vi "Crab.vi"   [LabVIEW 2020]
uses:
  Robot Global Data.vi
  <vilib>/addons/control/pid/pid.llb/PID (DBL).vi
  <vilib>/addons/control/pid/NI_PID_pid.lvlib
panel:
  # "p=0.014"
types:
  T1 = cluster{"proportional gain (Kc)":dbl, "integral time (Ti, min)":dbl, "derivative time (Td, min)":dbl}
  T2 = typedef "WPI_MotorControlDeviceRef.ctl" = cluster{"DeviceStatus":errorcluster, "Type":T3, "PWM":cluster{"PWM Channel":T4, "DeadBand":T5}, "CAN":cluster{"Device Number":u8, "SetOutput VI Ref":variant, "GetOutput VI Ref":variant, "Enable VI Ref":variant, "Disable VI Ref":variant, "Data":variant}, "Invert":bool, "DIO PWM":cluster{"PWM \"Enable\" Channel":T4, "DIOChannel":T6, "PWM Rate":dbl}}
  T3 = typedef "WPI_MotorControlType.ctl" = enum16{"PWM", "CAN", "DIO PWM"}
  T4 = typedef "FPGA_DIOPWMChannel.ctl" = enum8{"PWM 0", "PWM 1", "PWM 2", "PWM 3", "PWM 4", "PWM 5", "PWM 6", "PWM 7", "PWM 8", "PWM 9", "PWM MXP 0", "PWM MXP 1", "PWM MXP 2", "PWM MXP 3", "PWM MXP 4", "PWM MXP 5", "PWM MXP 6", "PWM MXP 7", "PWM MXP 8", "PWM MXP 9", "Invalid"}
  T5 = typedef "WPI_PWMDeadband.ctl" = cluster{"Name":string, "maxPositivePwm":i32, "minPositivePwm":i32, "centerPwm":i32, "maxNegativePwm":i32, "minNegativePwm":i32, "angularRange":u16}
  T6 = typedef "FPGA_DIOChannel.ctl" = enum8{"DIO 0", "DIO 1", "DIO 2", "DIO 3", "DIO 4", "DIO 5", "DIO 6", "DIO 7", "DIO 8", "DIO 9", "DIO MXP 0", "DIO MXP 1", "DIO MXP 2", "DIO MXP 3", "DIO MXP 4", "DIO MXP 5", "DIO MXP 6", "DIO MXP 7", "DIO MXP 8", "DIO MXP 9", "DIO MXP 10", "DIO MXP 11", "DIO MXP 12", "DIO MXP 13", "DIO MXP 14", "DIO MXP 15", "SPI Port CS1", "SPI Port CS2", "SPI Port CS3", "SPI Port MISO", "SPI Port MOSI", "Invalid"}
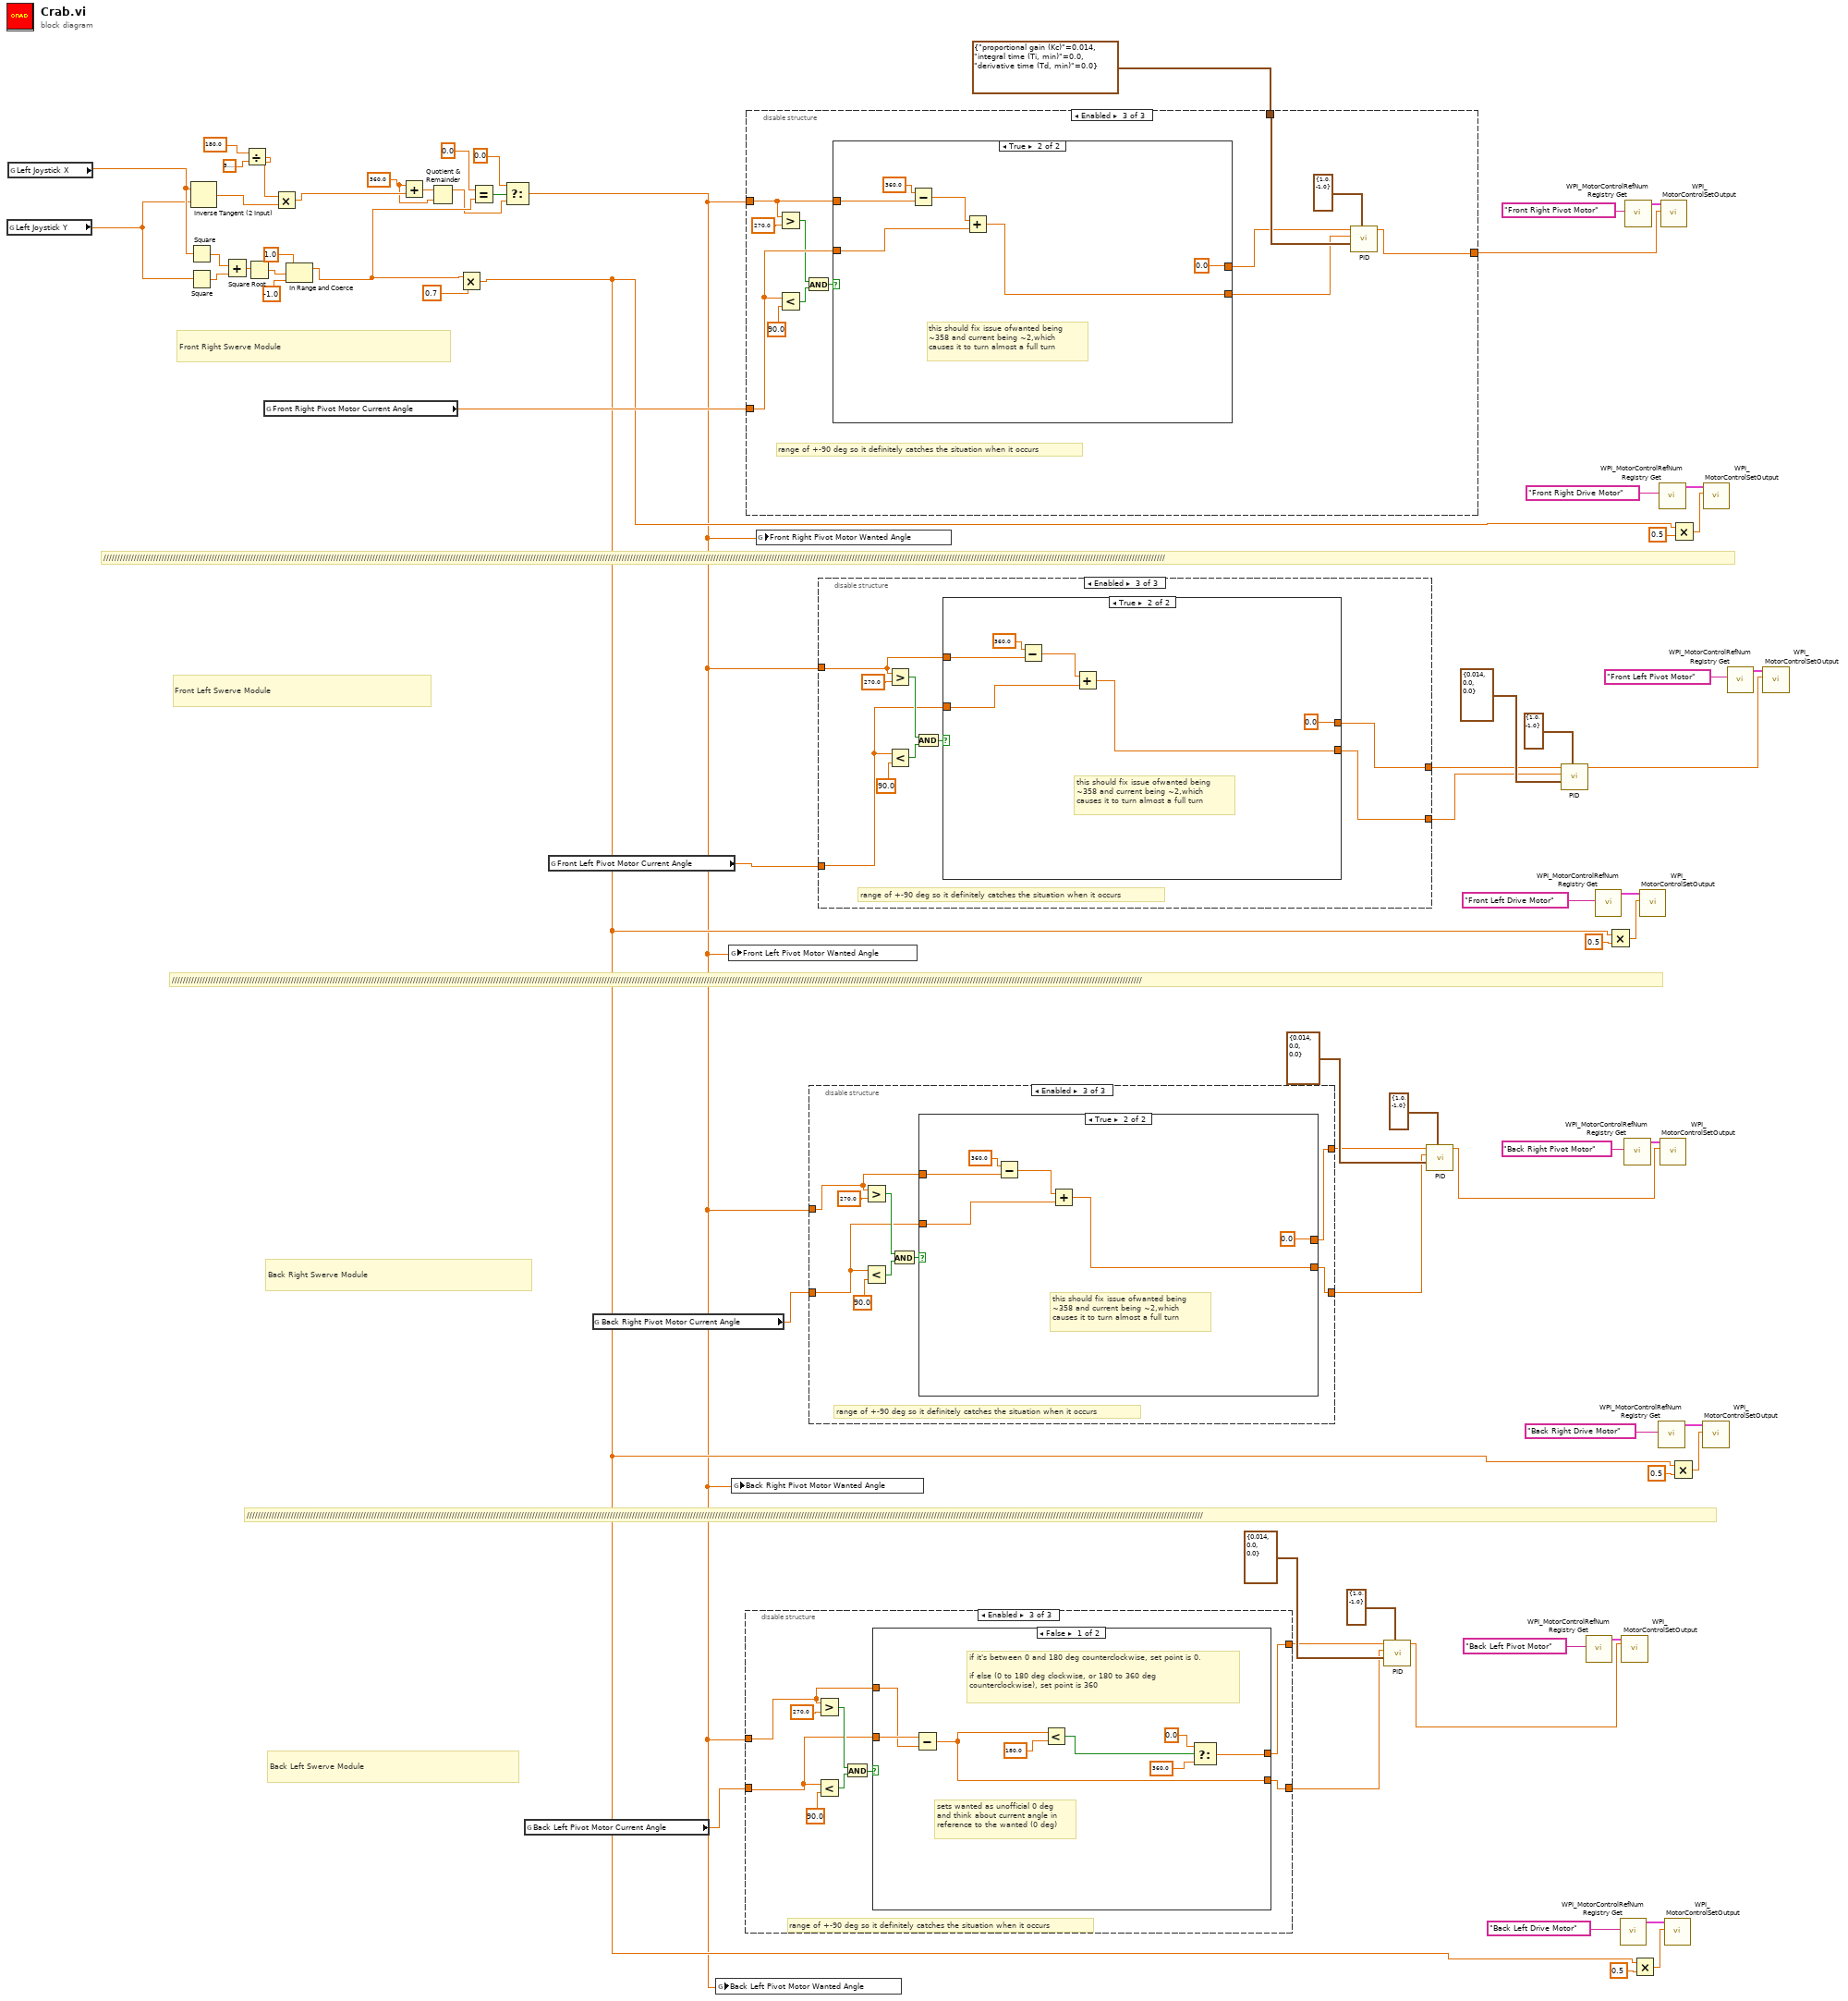
[diagram p0: block diagram]
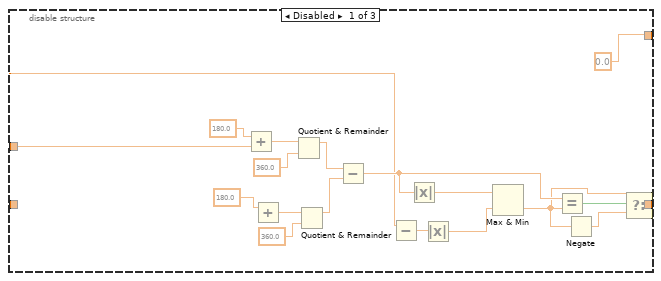
[diagram p2: hidden frame]
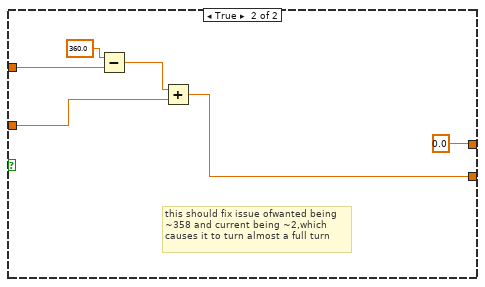
[diagram p4: hidden frame]
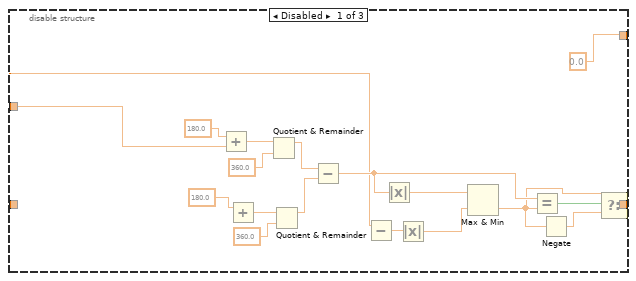
[diagram p5: hidden frame]
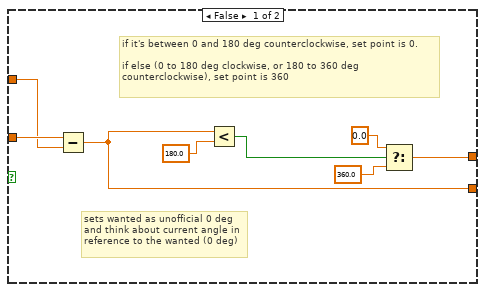
[diagram p7: hidden frame]
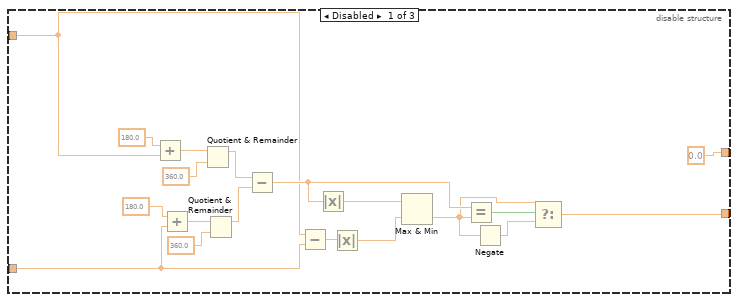
[diagram p8: hidden frame]
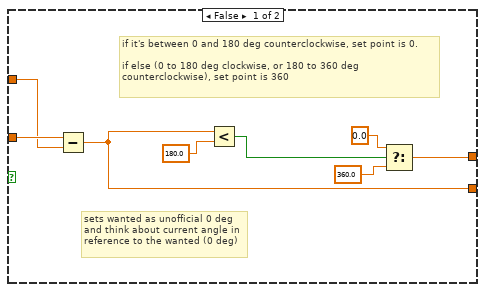
[diagram p10: hidden frame]
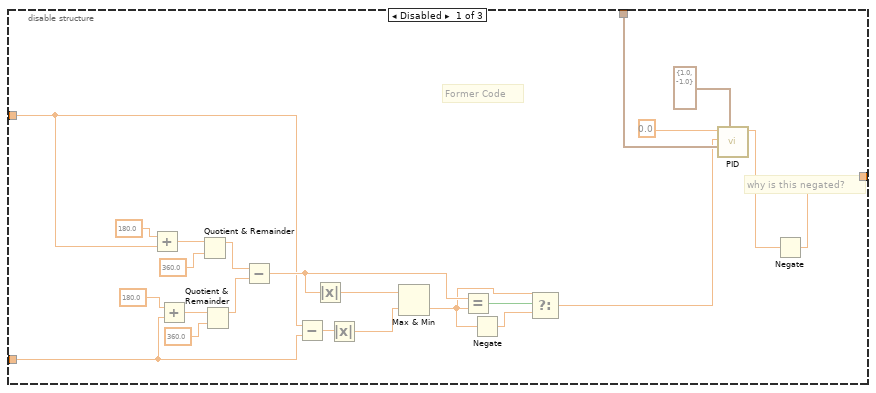
[diagram p11: hidden frame]
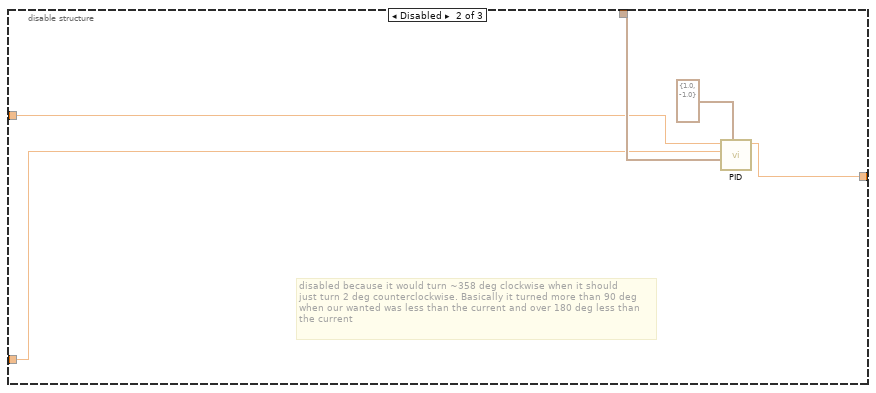
[diagram p12: hidden frame]
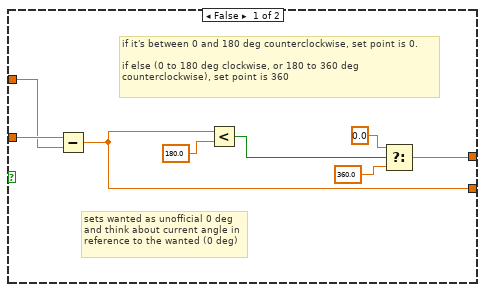
[diagram p13: hidden frame]
diagram:
  w60 = 360.0
  # "Back Left Swerve Module"
  # "/////////////////////////////////////////////////////////////////////////////////////////////////////////////////////////////////////////////////////////////////////////////////////////////////////////////////////////////////////////////////////////////////////////////////////////////////////////////////////////////////////////////////////////"
  # "//////////////////////////////////////////////////////////////////////////////////////////////////////////////////////////////////////////////////////////////////////////////////////////////////////////////////////////////////////////////////////////////////////////////////////////////////////////////////////////////////////////////////////////////"
  # "///////////////////////////////////////////////////////////////////////////////////////////////////////////////////////////////////////////////////////////////////////////////////////////////////////////////////////////////////////////////////////////////////////////////////////////////////////////////////////////////////////////////////////////////////////////////////////////////"
  # "Back Right Swerve Module"
  # "Front Left Swerve Module"
  # "Front Right Swerve Module"
  n1 = global read "Robot Global Data.vi" "Left Joystick Y"() -> (w50:dbl)
  n2 = global read "Robot Global Data.vi" "Left Joystick X"() -> (w51:dbl)
  n3 = Square(x=w51) -> (x^2=w57:dbl)
  n4 = Square(x=w50) -> (x^2=w56:dbl)
  n5 = Inverse Tangent (2 Input)(1:w50, 2:w51) -> (0:w55:dbl)
  n6 = Add(x=w57, y=w56) -> (x+y=w58:dbl)
  n7 = Divide(x=180.0, y=3.141592653589793) -> (x/y=w54:dbl)
  n8 = Square Root(x=w58) -> (sqrt(x)=w63:dbl)
  n9 = global read "Robot Global Data.vi" "Front Right Pivot Motor Current Angle"() -> (w26:dbl)
  n10 = Multiply(x=w54, y=w55) -> (x*y=w61:dbl)
  n11 = In Range and Coerce(upper limit=1.0, x=w63, lower limit=-1.0 ("upper limit")) -> (coerced(x)=w31:dbl)  [unwired: 1 out]
  n12 = Add(x=w60, y=w61) -> (x+y=w59:dbl)
  n13 = Quotient & Remainder(x=w59, y=w60) -> (x-y*floor(x/y)=w5:dbl)  [unwired: 1 out]
  n14 = Multiply(x=w31, y=0.7) -> (x*y=w6:dbl)
  n15 = Equal?(x=0.0, y=w31) -> (x = y?=w62:bool)
  n16 = Select(t=0.0, s=w62, f=w5) -> (s? t:f=w4:dbl)
  n17 = global read "Robot Global Data.vi" "Back Left Pivot Motor Current Angle"() -> (w7:dbl)
  n18 = global read "Robot Global Data.vi" "Front Left Pivot Motor Current Angle"() -> (w25:dbl)
  n19 = global read "Robot Global Data.vi" "Back Right Pivot Motor Current Angle"() -> (w19:dbl)
  n20 = global write "Robot Global Data.vi" "Back Left Pivot Motor Wanted Angle"(w4) -> ()
  n21 = global write "Robot Global Data.vi" "Front Left Pivot Motor Wanted Angle"(w4) -> ()
  n22 = global write "Robot Global Data.vi" "Back Right Pivot Motor Wanted Angle"(w4) -> ()
  n23 = disable-structure shown="Enabled" {
    disable-tunnel: w4 -> [w71 w88 w92]
    disable-tunnel: [w70 w87 w89] -> w10
    disable-tunnel: [0.0 w88 w90] -> w8
    disable-tunnel: w7 -> [_ w87 w91]
    frame Disabled {
      n24 = Add(x=180.0, y=w71) -> (x+y=w82:dbl)
      n25 = Add(x=180.0) -> (x+y=w80:dbl)  [unwired: 1 in]
      n26 = Quotient & Remainder(x=w82, y=360.0) -> (x-y*floor(x/y)=w78:dbl)  [unwired: 1 out]
      n27 = Quotient & Remainder(x=w80, y=360.0) -> (x-y*floor(x/y)=w77:dbl)  [unwired: 1 out]
      n28 = Subtract(x=w78, y=w77) -> (x-y=w76:dbl)
      n29 = Subtract(x=w71) -> (x-y=w75:dbl)  [unwired: 1 in]
      n30 = Absolute Value(x=w76) -> (abs(x)=w74:dbl)
      n31 = Absolute Value(x=w75) -> (abs(x)=w73:dbl)
      n32 = Max & Min(x=w74, y=w73) -> (min(x,y)=w72:dbl)  [unwired: 1 out]
      n33 = Equal?(x=w76, y=w72) -> (x = y?=w83:bool)
      n34 = Negate(x=w72) -> (-x=w84:dbl)
      n35 = Select(t=w72, s=w83, f=w84) -> (s? t:f=w70:dbl)
    }
    frame Disabled {
      # "disabled because it would turn ~358 deg clockwise when it should \njust turn 2 deg counterclockwise. Basically it turned more than 90 deg\nwhen our wanted was less than the current and over 180 deg less than\nthe current"
    }
    frame Enabled {
      # "range of +-90 deg so it definitely catches the situation when it occurs"
      n36 = Greater?(x=w92, y=270.0) -> (0:w93:bool)
      n37 = Less?(x=w91, y=90.0) -> (x < y?=w94:bool)
      n38 = And(x=w93, y=w94) -> (x .and. y?=w95:bool)
      n39 = case shown="False" w95 {
        tunnel: [w105 0.0] -> w90
        tunnel: w91 -> [w100 w108]
        tunnel: w92 -> [w99 w111]
        tunnel: [w98 w107] -> w89
        frame False {
          # "if it's between 0 and 180 deg counterclockwise, set point is 0.\n \nif else (0 to 180 deg clockwise, or 180 to 360 deg \ncounterclockwise), set point is 360"
          # "sets wanted as unofficial 0 deg\nand think about current angle in\nreference to the wanted (0 deg)"
          n40 = Subtract(x=w100, y=w99) -> (x-y=w98:dbl)
          n41 = Less?(x=w98, y=180.0 ("upper limit")) -> (x < y?=w104:bool)
          n42 = Select(t=0.0, s=w104, f=360.0) -> (s? t:f=w105:dbl)
        }
        frame True {
          # "this should fix issue ofwanted being\n~358 and current being ~2,which \ncauses it to turn almost a full turn"
          n43 = Subtract(x=360.0, y=w111) -> (x-y=w109:dbl)
          n44 = Add(x=w109, y=w108) -> (x+y=w107:dbl)
        }
      }
    }
  }
  n45 = disable-structure shown="Enabled" {
    disable-tunnel: T1 {"proportional gain (Kc)"=0.014, "integral time (Ti, min)"=0.0, "derivative time (Td, min)"=0.0} ("FR Pivot Motor PID gains") -> [w134 w138 w150]
    disable-tunnel: w26 -> [w131 w136 w144]
    disable-tunnel: w4 -> [w113 w137 w146]
    disable-tunnel: [w112 w135 w149] -> w22
    frame Disabled {
      # "why is this negated?"
      # "Former Code"
      n46 = Add(x=180.0, y=w113) -> (x+y=w125:dbl)
      n47 = Add(x=180.0, y=w131) -> (x+y=w123:dbl)
      n48 = Quotient & Remainder(x=w125, y=360.0) -> (x-y*floor(x/y)=w121:dbl)  [unwired: 1 out]
      n49 = Quotient & Remainder(x=w123, y=360.0) -> (x-y*floor(x/y)=w120:dbl)  [unwired: 1 out]
      n50 = Subtract(x=w121, y=w120) -> (x-y=w119:dbl)
      n51 = Subtract(x=w113, y=w131) -> (x-y=w118:dbl)
      n52 = Absolute Value(x=w119) -> (abs(x)=w117:dbl)
      n53 = Absolute Value(x=w118) -> (abs(x)=w116:dbl)
      n54 = Max & Min(x=w117, y=w116) -> (min(x,y)=w115:dbl)  [unwired: 1 out]
      n55 = Equal?(x=w119, y=w115) -> (x = y?=w126:bool)
      n56 = Negate(x=w115) -> (-x=w127:dbl)
      n57 = Select(t=w115, s=w126, f=w127) -> (s? t:f=w128:dbl)
      n58 = call-poly <vilib>:"PID.vi"("output range"=cluster{"output high":dbl, "output low":dbl} {"output high"=1.0, "output low"=-1.0}, "PID gains"=w134, "process variable"=w128, "setpoint"=0.0) -> ("output"=w114:dbl)  [unwired: 6 in, 1 out]
      n59 = Negate(x=w114) -> (-x=w112:dbl)
    }
    frame Disabled {
      # "disabled because it would turn ~358 deg clockwise when it should \njust turn 2 deg counterclockwise. Basically it turned more than 90 deg\nwhen our wanted was less than the current and over 180 deg less than\nthe current"
      n60 = call-poly <vilib>:"PID.vi"("output range"=cluster{"output high":dbl, "output low":dbl} {"output high"=1.0, "output low"=-1.0}, "PID gains"=w138, "process variable"=w136, "setpoint"=w137) -> ("output"=w135:dbl)  [unwired: 6 in, 1 out]
    }
    frame Enabled {
      # "range of +-90 deg so it definitely catches the situation when it occurs"
      n61 = Greater?(x=w146, y=270.0) -> (0:w140:bool)
      n62 = Less?(x=w144, y=90.0) -> (x < y?=w141:bool)
      n63 = And(x=w140, y=w141) -> (x .and. y?=w142:bool)
      n64 = case shown="True" w142 {
        tunnel: [w159 0.0] -> w148
        tunnel: w144 -> [w154 w162]
        tunnel: w146 -> [w153 w165]
        tunnel: [w152 w161] -> w147
        frame False {
          # "if it's between 0 and 180 deg counterclockwise, set point is 0.\n \nif else (0 to 180 deg clockwise, or 180 to 360 deg \ncounterclockwise), set point is 360"
          # "sets wanted as unofficial 0 deg\nand think about current angle in\nreference to the wanted (0 deg)"
          n65 = Subtract(x=w154, y=w153) -> (x-y=w152:dbl)
          n66 = Less?(x=w152, y=180.0 ("upper limit")) -> (x < y?=w158:bool)
          n67 = Select(t=0.0, s=w158, f=360.0) -> (s? t:f=w159:dbl)
        }
        frame True {
          # "this should fix issue ofwanted being\n~358 and current being ~2,which \ncauses it to turn almost a full turn"
          n68 = Subtract(x=360.0, y=w165) -> (x-y=w163:dbl)
          n69 = Add(x=w163, y=w162) -> (x+y=w161:dbl)
        }
      }
      n70 = call-poly <vilib>:"PID.vi"("output range"=cluster{"output high":dbl, "output low":dbl} {"output high"=1.0, "output low"=-1.0}, "PID gains"=w150, "process variable"=w147, "setpoint"=w148) -> ("output"=w149:dbl)  [unwired: 6 in, 1 out]
    }
  }
  n71 = global write "Robot Global Data.vi" "Front Right Pivot Motor Wanted Angle"(w4) -> ()
  n72 = disable-structure shown="Enabled" {
    disable-tunnel: w4 -> [w168 w185 w187]
    disable-tunnel: [w167 w184 w188] -> w24
    disable-tunnel: [0.0 w185 w189] -> w20
    disable-tunnel: w19 -> [_ w184 w186]
    frame Disabled {
      n73 = Add(x=180.0, y=w168) -> (x+y=w179:dbl)
      n74 = Add(x=180.0) -> (x+y=w177:dbl)  [unwired: 1 in]
      n75 = Quotient & Remainder(x=w179, y=360.0) -> (x-y*floor(x/y)=w175:dbl)  [unwired: 1 out]
      n76 = Quotient & Remainder(x=w177, y=360.0) -> (x-y*floor(x/y)=w174:dbl)  [unwired: 1 out]
      n77 = Subtract(x=w175, y=w174) -> (x-y=w173:dbl)
      n78 = Subtract(x=w168) -> (x-y=w172:dbl)  [unwired: 1 in]
      n79 = Absolute Value(x=w173) -> (abs(x)=w171:dbl)
      n80 = Absolute Value(x=w172) -> (abs(x)=w170:dbl)
      n81 = Max & Min(x=w171, y=w170) -> (min(x,y)=w169:dbl)  [unwired: 1 out]
      n82 = Equal?(x=w173, y=w169) -> (x = y?=w180:bool)
      n83 = Negate(x=w169) -> (-x=w181:dbl)
      n84 = Select(t=w169, s=w180, f=w181) -> (s? t:f=w167:dbl)
    }
    frame Disabled {
      # "disabled because it would turn ~358 deg clockwise when it should \njust turn 2 deg counterclockwise. Basically it turned more than 90 deg\nwhen our wanted was less than the current and over 180 deg less than\nthe current"
    }
    frame Enabled {
      # "range of +-90 deg so it definitely catches the situation when it occurs"
      n85 = Greater?(x=w187, y=270.0) -> (0:w190:bool)
      n86 = Less?(x=w186, y=90.0) -> (x < y?=w191:bool)
      n87 = And(x=w190, y=w191) -> (x .and. y?=w192:bool)
      n88 = case shown="True" w192 {
        tunnel: [w202 0.0] -> w189
        tunnel: w186 -> [w197 w205]
        tunnel: w187 -> [w196 w208]
        tunnel: [w195 w204] -> w188
        frame False {
          # "if it's between 0 and 180 deg counterclockwise, set point is 0.\n \nif else (0 to 180 deg clockwise, or 180 to 360 deg \ncounterclockwise), set point is 360"
          # "sets wanted as unofficial 0 deg\nand think about current angle in\nreference to the wanted (0 deg)"
          n89 = Subtract(x=w197, y=w196) -> (x-y=w195:dbl)
          n90 = Less?(x=w195, y=180.0 ("upper limit")) -> (x < y?=w201:bool)
          n91 = Select(t=0.0, s=w201, f=360.0) -> (s? t:f=w202:dbl)
        }
        frame True {
          # "this should fix issue ofwanted being\n~358 and current being ~2,which \ncauses it to turn almost a full turn"
          n92 = Subtract(x=360.0, y=w208) -> (x-y=w206:dbl)
          n93 = Add(x=w206, y=w205) -> (x+y=w204:dbl)
        }
      }
    }
  }
  n94 = disable-structure shown="Enabled" {
    disable-tunnel: w25 -> [w212 w228 w230]
    disable-tunnel: [w211 w228 w233] -> w1
    disable-tunnel: w4 -> [w210 w229 w231]
    disable-tunnel: [0.0 w229 w232] -> w2
    frame Disabled {
      n95 = Add(x=180.0, y=w210) -> (x+y=w223:dbl)
      n96 = Add(x=180.0, y=w212) -> (x+y=w221:dbl)
      n97 = Quotient & Remainder(x=w223, y=360.0) -> (x-y*floor(x/y)=w219:dbl)  [unwired: 1 out]
      n98 = Quotient & Remainder(x=w221, y=360.0) -> (x-y*floor(x/y)=w218:dbl)  [unwired: 1 out]
      n99 = Subtract(x=w219, y=w218) -> (x-y=w217:dbl)
      n100 = Subtract(x=w210, y=w212) -> (x-y=w216:dbl)
      n101 = Absolute Value(x=w217) -> (abs(x)=w215:dbl)
      n102 = Absolute Value(x=w216) -> (abs(x)=w214:dbl)
      n103 = Max & Min(x=w215, y=w214) -> (min(x,y)=w213:dbl)  [unwired: 1 out]
      n104 = Equal?(x=w217, y=w213) -> (x = y?=w224:bool)
      n105 = Negate(x=w213) -> (-x=w225:dbl)
      n106 = Select(t=w213, s=w224, f=w225) -> (s? t:f=w211:dbl)
    }
    frame Disabled {
      # "disabled because it would turn ~358 deg clockwise when it should \njust turn 2 deg counterclockwise. Basically it turned more than 90 deg\nwhen our wanted was less than the current and over 180 deg less than\nthe current"
    }
    frame Enabled {
      # "range of +-90 deg so it definitely catches the situation when it occurs"
      n107 = Greater?(x=w231, y=270.0) -> (0:w234:bool)
      n108 = Less?(x=w230, y=90.0) -> (x < y?=w235:bool)
      n109 = And(x=w234, y=w235) -> (x .and. y?=w236:bool)
      n110 = case shown="True" w236 {
        tunnel: [w246 0.0] -> w232
        tunnel: w230 -> [w241 w249]
        tunnel: w231 -> [w240 w252]
        tunnel: [w239 w248] -> w233
        frame False {
          # "if it's between 0 and 180 deg counterclockwise, set point is 0.\n \nif else (0 to 180 deg clockwise, or 180 to 360 deg \ncounterclockwise), set point is 360"
          # "sets wanted as unofficial 0 deg\nand think about current angle in\nreference to the wanted (0 deg)"
          n111 = Subtract(x=w241, y=w240) -> (x-y=w239:dbl)
          n112 = Less?(x=w239, y=180.0 ("upper limit")) -> (x < y?=w245:bool)
          n113 = Select(t=0.0, s=w245, f=360.0) -> (s? t:f=w246:dbl)
        }
        frame True {
          # "this should fix issue ofwanted being\n~358 and current being ~2,which \ncauses it to turn almost a full turn"
          n114 = Subtract(x=360.0, y=w252) -> (x-y=w250:dbl)
          n115 = Add(x=w250, y=w249) -> (x+y=w248:dbl)
        }
      }
    }
  }
  n116 = call-poly <vilib>:"PID.vi"("output range"=cluster{"output high":dbl, "output low":dbl} {"output high"=1.0, "output low"=-1.0}, "PID gains"=T1 {"proportional gain (Kc)"=0.014, "integral time (Ti, min)"=0.0, "derivative time (Td, min)"=0.0} ("FR Pivot Motor PID gains"), "process variable"=w10, "setpoint"=w8) -> ("output"=w9:dbl)  [unwired: 6 in, 1 out]
  n117 = call-poly <vilib>:"PID.vi"("output range"=cluster{"output high":dbl, "output low":dbl} {"output high"=1.0, "output low"=-1.0}, "PID gains"=T1 {"proportional gain (Kc)"=0.014, "integral time (Ti, min)"=0.0, "derivative time (Td, min)"=0.0} ("FR Pivot Motor PID gains"), "process variable"=w24, "setpoint"=w20) -> ("output"=w23:dbl)  [unwired: 6 in, 1 out]
  n118 = call-poly <vilib>:"PID.vi"("output range"=cluster{"output high":dbl, "output low":dbl} {"output high"=1.0, "output low"=-1.0}, "PID gains"=T1 {"proportional gain (Kc)"=0.014, "integral time (Ti, min)"=0.0, "derivative time (Td, min)"=0.0} ("FR Pivot Motor PID gains"), "process variable"=w1, "setpoint"=w2) -> ("output"=w21:dbl)  [unwired: 6 in, 1 out]
  n119 = call <vilib>:"WPI_MotorControlRefNum Registry Get.vi"("refnum name"="Back Left Pivot Motor") -> ("MotorControlDevRef"=w17:T2)  [unwired: 9 in, 1 out]
  n120 = call <vilib>:"WPI_MotorControlRefNum Registry Get.vi"("refnum name"="Front Left Drive Motor") -> ("MotorControlDevRef"=w43:T2)  [unwired: 9 in, 1 out]
  n121 = Multiply(x=w6, y=0.5) -> (x*y=w41:dbl)
  n122 = call <vilib>:"WPI_MotorControlRefNum Registry Get.vi"("refnum name"="Back Left Drive Motor") -> ("MotorControlDevRef"=w16:T2)  [unwired: 9 in, 1 out]
  n123 = call <vilib>:"WPI_MotorControlSetOutput.vi"("Output"=w9, "MotorControlDevRef"=w17) -> ()  [unwired: 7 in, 3 out]
  n124 = call <vilib>:"WPI_MotorControlRefNum Registry Get.vi"("refnum name"="Back Right Pivot Motor") -> ("MotorControlDevRef"=w38:T2)  [unwired: 9 in, 1 out]
  n125 = call <vilib>:"WPI_MotorControlRefNum Registry Get.vi"("refnum name"="Front Right Pivot Motor") -> ("MotorControlDevRef"=w67:T2)  [unwired: 9 in, 1 out]
  n126 = Multiply(x=w6, y=0.5) -> (x*y=w14:dbl)
  n127 = call <vilib>:"WPI_MotorControlSetOutput.vi"("Output"=w41, "MotorControlDevRef"=w43) -> ()  [unwired: 7 in, 3 out]
  n128 = call <vilib>:"WPI_MotorControlRefNum Registry Get.vi"("refnum name"="Back Right Drive Motor") -> ("MotorControlDevRef"=w37:T2)  [unwired: 9 in, 1 out]
  n129 = call <vilib>:"WPI_MotorControlRefNum Registry Get.vi"("refnum name"="Front Right Drive Motor") -> ("MotorControlDevRef"=w49:T2)  [unwired: 9 in, 1 out]
  n130 = call <vilib>:"WPI_MotorControlSetOutput.vi"("Output"=w23, "MotorControlDevRef"=w38) -> ()  [unwired: 7 in, 3 out]
  n131 = call <vilib>:"WPI_MotorControlSetOutput.vi"("Output"=w22, "MotorControlDevRef"=w67) -> ()  [unwired: 7 in, 3 out]
  n132 = call <vilib>:"WPI_MotorControlSetOutput.vi"("Output"=w14, "MotorControlDevRef"=w16) -> ()  [unwired: 7 in, 3 out]
  n133 = Multiply(x=w6, y=0.5) -> (x*y=w35:dbl)
  n134 = Multiply(x=w6, y=0.5) -> (x*y=w47:dbl)
  n135 = call <vilib>:"WPI_MotorControlSetOutput.vi"("Output"=w35, "MotorControlDevRef"=w37) -> ()  [unwired: 7 in, 3 out]
  n136 = call <vilib>:"WPI_MotorControlSetOutput.vi"("Output"=w47, "MotorControlDevRef"=w49) -> ()  [unwired: 7 in, 3 out]
  n137 = call <vilib>:"WPI_MotorControlRefNum Registry Get.vi"("refnum name"="Front Left Pivot Motor") -> ("MotorControlDevRef"=w44:T2)  [unwired: 9 in, 1 out]
  n138 = call <vilib>:"WPI_MotorControlSetOutput.vi"("Output"=w21, "MotorControlDevRef"=w44) -> ()  [unwired: 7 in, 3 out]
